vi "Generate Shipping List.vi"(8 "error in (no error)":errorcluster, 10 "Shipping ID":i32, 11 "Delivery in":refnum<class "Delivery.lvclass">) -> (0 "error out":errorcluster, 3 "Delivery out":refnum<class "Delivery.lvclass">)   [LabVIEW 2019, in "Delivery.lvclass"]
uses:
  Delivery.lvclass
panel:
  out "Price:":string
  out "Estimated Delivery Time:":string
  out "Transport Company:":string
  out "Parcel Delivery Address":string
  out "Parcel Pickup Address":string
  out "Shipping List ID:":string
  out "Recipient:":string
  in  "Stop":bool
  out "Sender:":string
  # "Shipping List"
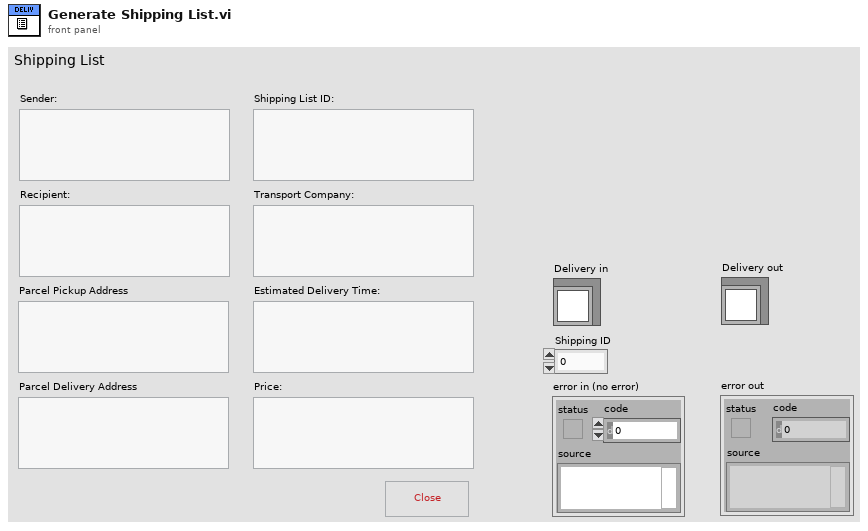
[diagram p1: front panel]
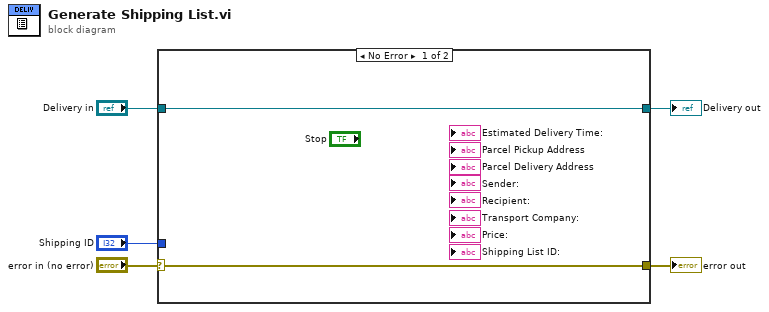
[diagram p0: block diagram]
diagram:
  n1 = case shown="No Error" "error in (no error)" {
    selector: "error in (no error)" -> [w6 w9]
    tunnel: [w6 w9] -> w4
    tunnel: [w7 w8] -> w2
    tunnel: "Delivery in" -> [w7 w8]
    tunnel: "Shipping ID" -> [_ _]
    frame No Error {
    }
    frame Error {
    }
  }
  "error out" <- w4
  "Delivery out" <- w2
